vi "Periodic Tasks.vi"(8 "error in (no error)":errorcluster) -> ()   [LabVIEW 2017]
doc: "This VI runs in parallel to other tasks. It can contain as many user-defined periodic loops as you need. These can carry out PID or other sorts of timed response."
panel:
  in  "Tab Control":T1(tab)
  out "PID Tracking Lift":T2(graph)
  out "Current Error Lift":dbl
  out "PID Tracking Arm":T2(graph)
  out "Current Error Arm":dbl
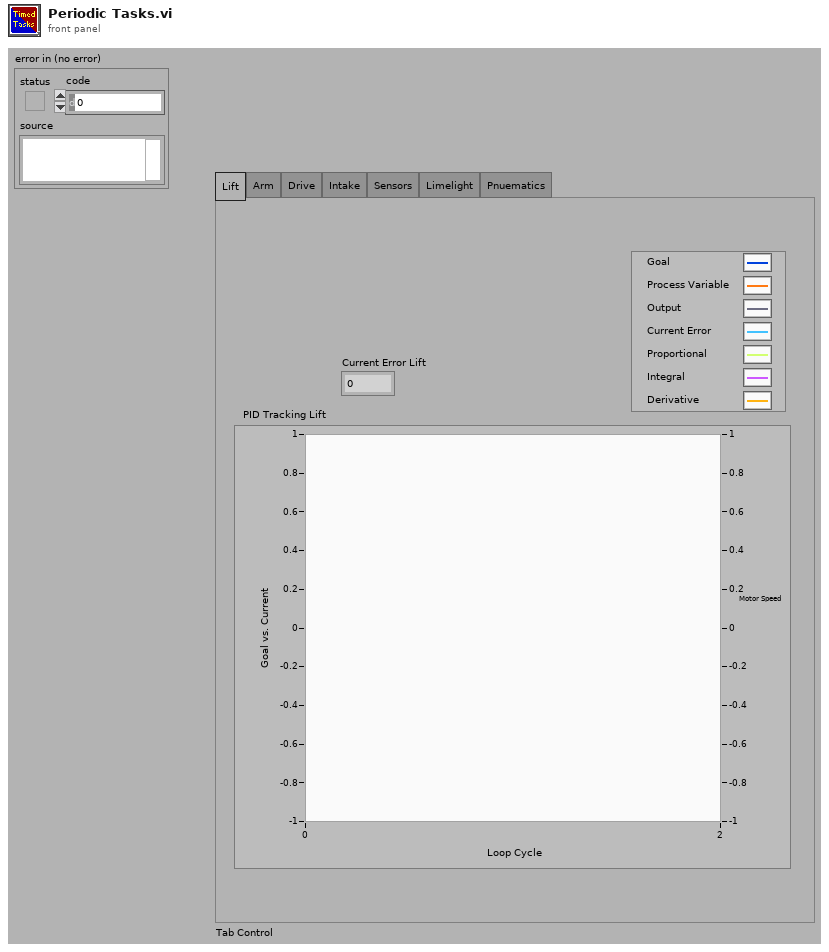
[diagram p1: front panel]
types:
  T1 = enum32{"Lift", "Arm", "Drive", "Intake", "Sensors", "Limelight", "Pnuematics"}
  T2 = cluster{"Goal":dbl, "Process Variable":dbl, "Max Ouput":dbl, dbl, dbl, dbl, dbl}
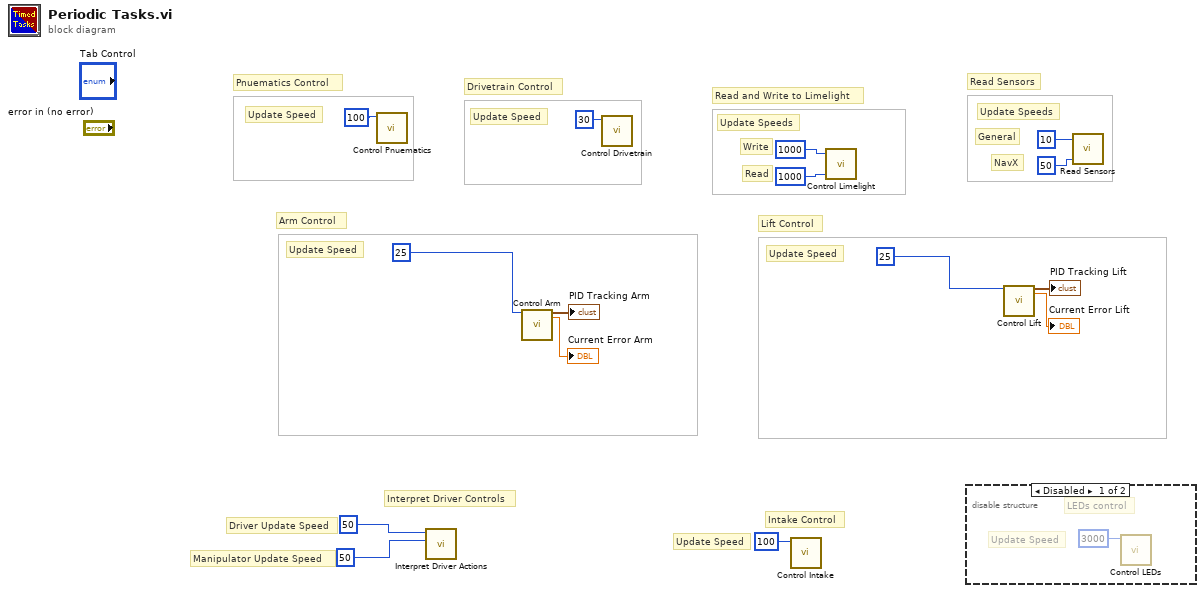
[diagram p0: block diagram]
diagram:
  # "Intake Control"
  # "Update Speed"
  # "Manipulator Update Speed"
  # "Driver Update Speed"
  # "Interpret Driver Controls"
  # "Update Speed"
  # "Update Speed"
  # "Update Speeds"
  # "NavX"
  # "General"
  # "Read Sensors"
  # "Pnuematics Control"
  # "Update Speed"
  # "Lift Control"
  # "Arm Control"
  # "Drivetrain Control"
  # "Update Speed"
  # "Read and Write to Limelight"
  # "Update Speeds"
  # "Read"
  # "Write"
  n1 = call "Control Pnuematics.vi"("Loop Time (ms)"=u32 100 ("Loop Timer (ms)")) -> ()  [unwired: 11 in]
  n2 = call "Interpret Driver Actions.vi"("loop time manipulator (ms)"=u32 50, "loop time driver (ms)"=u32 50 ("loop time (ms)")) -> ()  [unwired: 10 in]
  n3 = call "Control Arm.vi"("Loop Time (ms)"=u32 25) -> ("PID Tracking Arm"=→"PID Tracking Arm":T2, "Current Error Arm"=→"Current Error Arm":dbl)  [unwired: 17 in]
  n4 = call "Control Drivetrain.vi"("Loop Time (ms)"=u32 30) -> ()  [unwired: 11 in]
  n5 = call "Control Intake.vi"("loop time (ms)"=u32 100) -> ()  [unwired: 11 in]
  n6 = call "Control Limelight.vi"("Read Data Loop Time (ms) (min 10)"=u32 1000, "Write Data Loop Time (ms)"=u32 1000) -> ()  [unwired: 1 in]
  n7 = disable-structure shown="Disabled" {
    frame Disabled {
      # "LEDs control"
      # "Update Speed"
      n8 = call "Control LEDs.vi"("loop time (ms)"=u32 3000) -> ()  [unwired: 11 in]
    }
    frame Enabled {
    }
  }
  n9 = call "Control Lift.vi"("Loop Time (ms)"=u32 25) -> ("PID Tracking Lift Up"=→"PID Tracking Lift":T2, "Current Error Lift"=→"Current Error Lift":dbl)  [unwired: 17 in]
  n10 = call "Read Sensors.vi"("NavX Loop Time (ms)"=u32 50 ("Read Data Loop Time (ms) (min 10)"), "General Loop Time (ms)"=u32 10 ("Write Data Loop Time (ms)")) -> ()  [unwired: 1 in]
